vi "TextBoxLogCtrlMgr.Initialize.vi"(4 "DataStamp":bool, 6 "TimeStamp":bool=TRUE, 7 "MaxLen":i32=10000, 8 "error in (no error)":errorcluster, 9 "Auto Scroll":bool=TRUE, 10 "CtrlRef":refnum<vi>, 11 "TextBoxLogCtrlMgr in":refnum<class "TextBoxLogCtrlMgr.lvclass">) -> (0 "error out":errorcluster, 3 "TextBoxLogCtrlMgr out":refnum<class "TextBoxLogCtrlMgr.lvclass">)   [LabVIEW 2024, in "EQMF.lvlib" / "String Utils.lvlib" / "TextBoxLogCtrlMgr.lvclass"]
uses:
  TextBoxLogCtrlMgr.lvclass
  TextBoxLogCtrlMgr.lvclass/TextBoxLogCtrlMgr.ctl
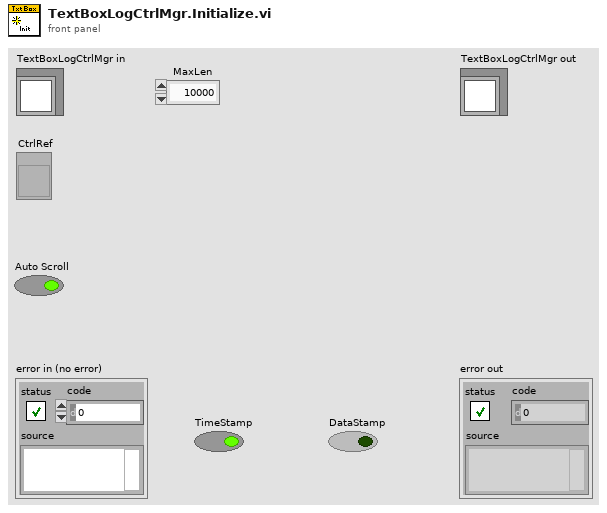
[diagram p1: front panel]
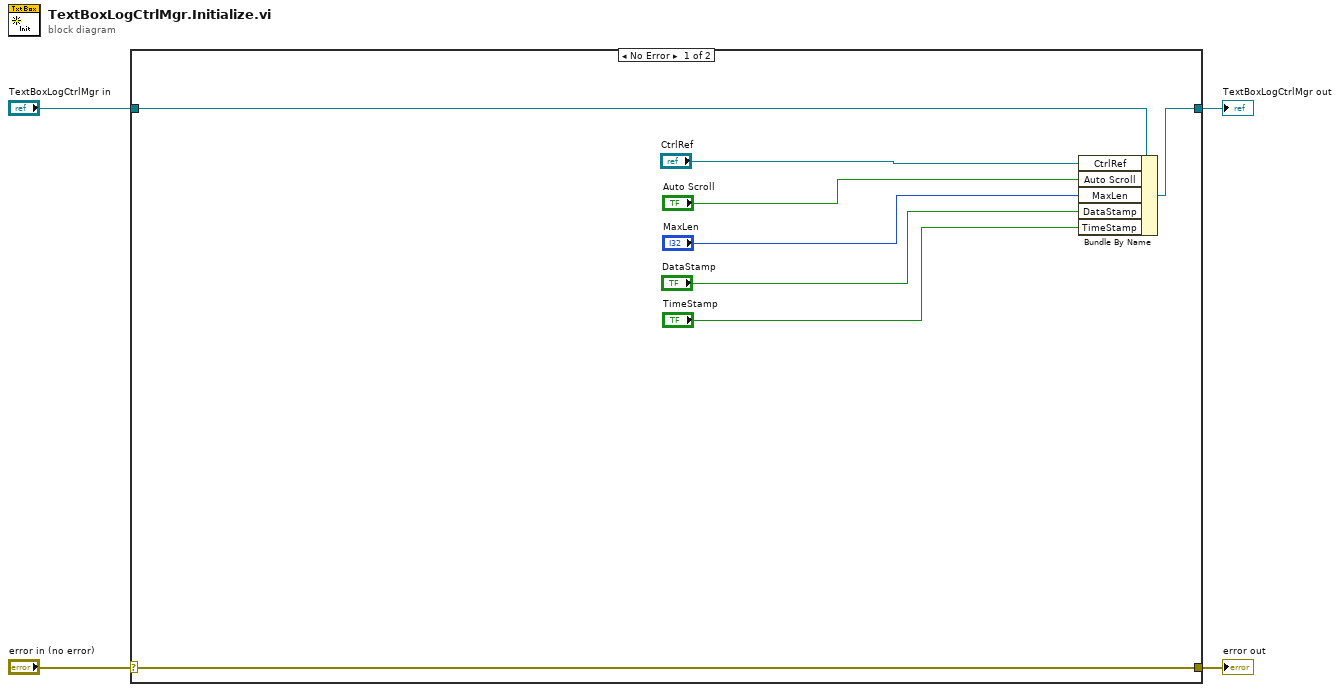
[diagram p0: block diagram]
diagram:
  n1 = case shown="No Error" "error in (no error)" {
    selector: "error in (no error)" -> [w12 w14]
    tunnel: [w12 w14] -> w3
    tunnel: [w11 w13] -> w1
    tunnel: "TextBoxLogCtrlMgr in" -> [w10 w13]
    frame No Error {
      n2 = Bundle By Name(cluster=w10, "CtrlRef"="CtrlRef", "Auto Scroll"="Auto Scroll", "MaxLen"="MaxLen", "DataStamp"="DataStamp", "TimeStamp"="TimeStamp") -> (w11:refnum<class "TextBoxLogCtrlMgr.lvclass">)
    }
    frame Error {
    }
  }
  "error out" <- w3
  "TextBoxLogCtrlMgr out" <- w1
